vi "NR_DeFreData .vi"(0 "appended path":path, 5 "Nsym_slot,":dbl, 7 "Nu":dbl, 9 "rxdata":cdb[](array[numeric]), 11 "error in (no error)":errorcluster caption="错误输入（无错误）", 12 "EN_TIMEOFFSETCP":dbl, 13 "timeoffsetCP":dbl) -> (1 "defredata":cdb[](array[numeric]), 14 "error IO":errorcluster)   [LabVIEW 2015]
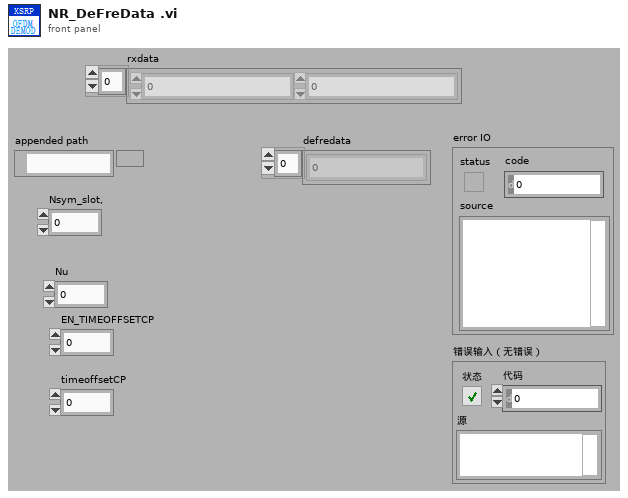
[diagram p1: front panel]
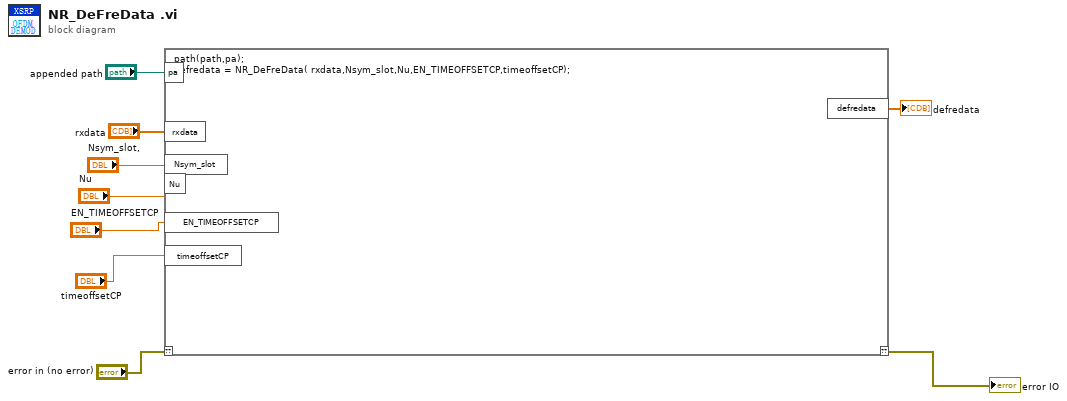
[diagram p0: block diagram]
diagram:
  n1 = script code="path(path,pa);\ndefredata = NR_DeFreData( rxdata,Nsym_slot,Nu,EN_TIMEOFFSETCP,timeoffsetCP);"("??"="error in (no error)", "pa"="appended path", "rxdata"="rxdata", "Nsym_slot"="Nsym_slot,", "Nu"="Nu", "EN_TIMEOFFSETCP"="EN_TIMEOFFSETCP", "timeoffsetCP"="timeoffsetCP") -> ("??"=→"error IO":errorcluster, "defredata"=→"defredata":cdb[])
